vi "Read NumberOfRobots.vi"(8 "error in (no error)":errorcluster, 11 "PrepareKeeperPassPlay in":refnum<class "PrepareKeeperPassPlay.lvclass">) -> (0 "error out":errorcluster, 2 "NumberOfRobots":dbl=2.0, 3 "PrepareKeeperPassPlay out":refnum<class "PrepareKeeperPassPlay.lvclass">)   [LabVIEW 2023, in "PrepareKeeperPassPlay.lvclass"]
uses:
  PrepareKeeperPassPlay.lvclass
  PrepareKeeperPassPlay.lvclass/PrepareKeeperPassPlay.ctl
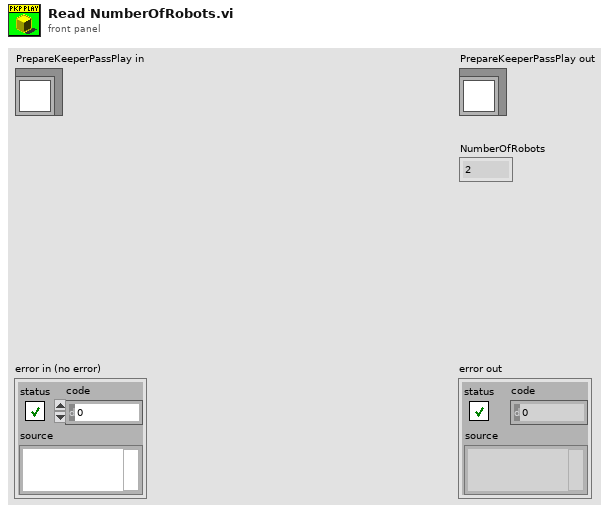
[diagram p1: front panel]
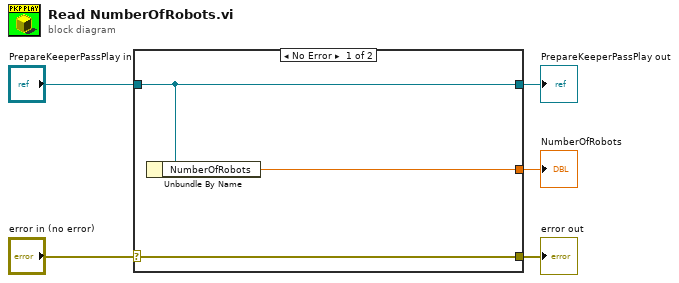
[diagram p0: block diagram]
diagram:
  n1 = case shown="No Error" "error in (no error)" {
    selector: "error in (no error)" -> [w8 w9]
    tunnel: [w8 w9] -> w4
    tunnel: [w7 w10] -> w2
    tunnel: "PrepareKeeperPassPlay in" -> [w7 w10]
    tunnel: [w6 _] -> w1
    frame No Error {
      n2 = Unbundle By Name(w7) -> ("NumberOfRobots"=w6:dbl)
    }
    frame Error {
    }
  }
  "error out" <- w4
  "PrepareKeeperPassPlay out" <- w2
  "NumberOfRobots" <- w1
